vi "ClusterEscala.vi"() -> ()   [LabVIEW 2020]
panel:
  out "Medidores":T1 {"Tank" scale=0.0..10.0; "Gauge" scale=0.0..10.0; "Thermometer" scale=0.0..100.0}
  in  "Controladores":T2
  out "x*y 2":cluster{dbl, dbl, dbl}
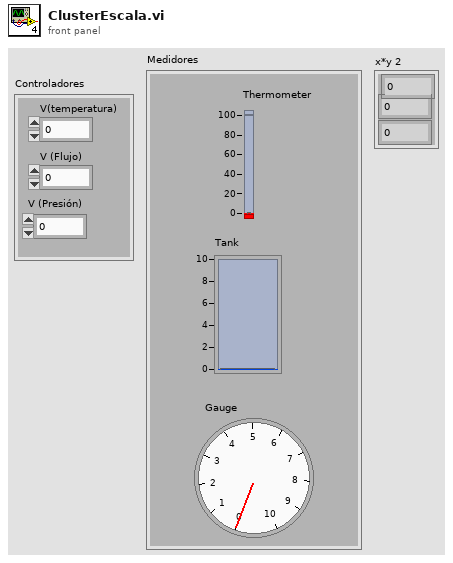
[diagram p1: front panel]
types:
  T1 = cluster{"Thermometer":dbl, "Tank":dbl, "Gauge":dbl}
  T2 = cluster{"V(temperatura)":dbl, "V (Flujo)":dbl, "V (Presión)":dbl}
  T3 = cluster{"°C/V":dbl, "(I/seg)/V":dbl, "(N/m^2)/V":dbl}
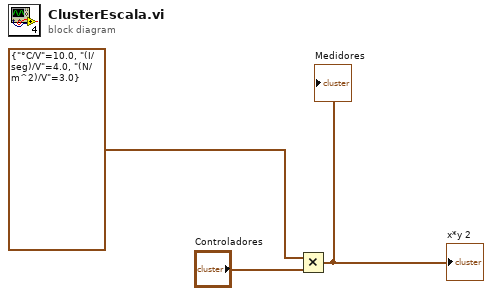
[diagram p0: block diagram]
diagram:
  n1 = Multiply(x=T3 {"°C/V"=10.0, "(I/seg)/V"=4.0, "(N/m^2)/V"=3.0}, y="Controladores") -> (x*y=→"x*y 2" →"Medidores":cluster{dbl, dbl, dbl})
